vi "CursorVolte.vi"(8 "Enable":bool, 9 "Volte":dbl, 10 "XYGraphUp":refnum<vi>, 11 "XYGraphDown":refnum<vi>) -> ()   [LabVIEW 2017]
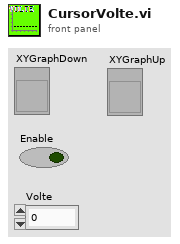
[diagram p1: front panel]
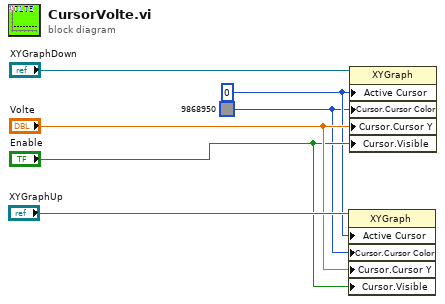
[diagram p0: block diagram]
diagram:
  w1 = u32 9868950
  w2 = u32 0 ("Active Cursor")
  n1 = property class="XYGraph"(reference="XYGraphUp", "Active Cursor"=w2, "Cursor.Cursor Color"=w1, "Cursor.Cursor Y"="Volte", "Cursor.Visible"="Enable") -> ()  [unwired: 1 in, 2 out]
  n2 = property class="XYGraph"(reference="XYGraphDown", "Active Cursor"=w2, "Cursor.Cursor Color"=w1, "Cursor.Cursor Y"="Volte", "Cursor.Visible"="Enable") -> ()  [unwired: 1 in, 2 out]
